vi "HOST_Demodulation_Array.vi"() -> ()   [LabVIEW 2020]
uses:
  <vilib>/rvi/interface/nirviMethod/nirviMethod.xnode
  <vilib>/rvi/errors/niLvFpgaMergeErrorWithErrorCode.vi
  <instrlib>/_niInstr/Streaming/v1/Host/niInstr Streaming v1 Host.lvlib
  <vilib>/rvi/interface/nirviReadWriteControl/nirviReadWriteControl.xnode
  <vilib>/rvi/interface/nirviCloseFPGA/nirviCloseFPGA.xnode
  <vilib>/rvi/interface/nirviOpenFPGA/nirviOpenFPGA.xnode
  <vilib>/rvi/interface/Simulation/niFpgaSimulationCallBeginRW.vi
  <vilib>/rvi/errors/niLvFpgaAdjustHostInterfaceError.vi
  <instrlib>/_niInstr/Streaming/v1/Host/Public/Wait for Stream.vi
  <instrlib>/_niInstr/Streaming/v1/Host/Public/Start Finite Stream.vi
  <instrlib>/_niInstr/Streaming/v1/Host/Public/Start Continuous Stream.vi
  FPGA Bitfiles/rfsignal_FPGATarget_ARRAYCOMPLETECOD_BYxh9E+ljbY.lvbitx
  <vilib>/FPGAPlugInAG/PXIe-7972R/niLvFpga_Open_PXIe-7972R.vi
  <vilib>/rvi/interface/common/dynamic/niFpgaDynamicAddResources.vi
  <vilib>/FPGAPlugInAG/Dynamic/niLvFpga_ConfigureFifo_Dynamic.vi
  <vilib>/FPGAPlugInAG/Dynamic/niLvFpga_StartFifo_Dynamic.vi
  <vilib>/FPGAPlugInAG/Dynamic/niLvFpga_WriteFifo_Dynamic.vi
  <vilib>/FPGAPlugInAG/Dynamic/niLvFpga_Close_Dynamic.vi
  <vilib>/userDefined/Silver/nirio_resource_slv.ctl
  Controls/Clock Select.ctl
panel:
  out "Feedback value check":fxp<+/-,48,32> format="%.26g"
  in  "Decimate AI":u16=100
  in  "CIC length":u16[](array[numeric])
  in  "CIC Cascades":enum16{"1 stage", "2 stage"}(ring)
  in  "Demod Phase 1":u32
  in  "demod":bool
  in  "Modulation":bool[](array[boolean])=[TRUE, FALSE, FALSE, FALSE, FALSE, FALSE, FALSE, FALSE]
  in  "Mod Amp":fxp<+,16,1>[](array[numeric])=[0.5, 1.0, 1.0, 1.0, 0.5, 1.0, 1.0, 1.0]
  in  "Mod Fq (MHz)":dbl[](array[numeric])=[0.1, 1.0, 1.0, 1.0, 0.1, 1.0, 0.0, 1.0] format="%5p"
  in  "stop":bool
  in  "Gain (multiplicative)":fxp<+,32,4>[](array[numeric])=[1.0, 1.0, 1.0, 1.0, 1.0, 1.0, 1.0, 1.0]
  in  "Wave Reader":dbl[](array[numeric])=[27000000.0, 27000000.0, 27000000.0, 27000000.0, 100.0, 27000000.0, 27000000.0, 27000000.0] format="%5p"
  out "AO":waveform(dbl)(graph)={"t0"=timestamp(0.0013999999999999998 s since 1904-01-01), "dt"=3.3333333333333334e-09, "Y"=array[60000 elements]}
  in  "Wave On":bool[](array[boolean])=[FALSE, FALSE, FALSE, FALSE, FALSE, FALSE, FALSE, FALSE]
  in  "Amplitude (V)":dbl[](array[numeric])=[0.33, 0.1, 0.12, 0.12, 0.33, 0.12, 0.12, 0.12] format="%0.2p"
  in  "Frequencies (Hz)":dbl[](array[numeric])=[20000.0, 20000.0, 20000.0, 20000.0, 20000.0, 20000.0, 20000.0, 20000.0] format="%5.0p"
  in  "Signal Type":T1(ring)
  in  "Sampling Info":cluster{"Fs":dbl, "#s":dbl}={"Fs"=300000000.0, "#s"=60000.0} {"Fs" format="%#_3p"}
  out "Error Out":errorcluster
  in  "Update Waveform":bool
  in  "AO Channel":T2(ring)
  in  "Clock Select":T3 items=["Internal Clock", "Internal Clock w/ Ref via CLK/REF IN", "Internal Clock w/ Ref via Sync Clock", "External Clock via CLK/REF IN"]
  in  "Rate of External Sample Clock (MHz)":u16=100 min=60 max=100 step=1
  in  "RIO Resource":T4="RIO0"
  # "Analog In"
  # "Waveform Modification"
  # "Waveform Initialization"
  # "CH1"
  # "Don't change"
  # "CH2"
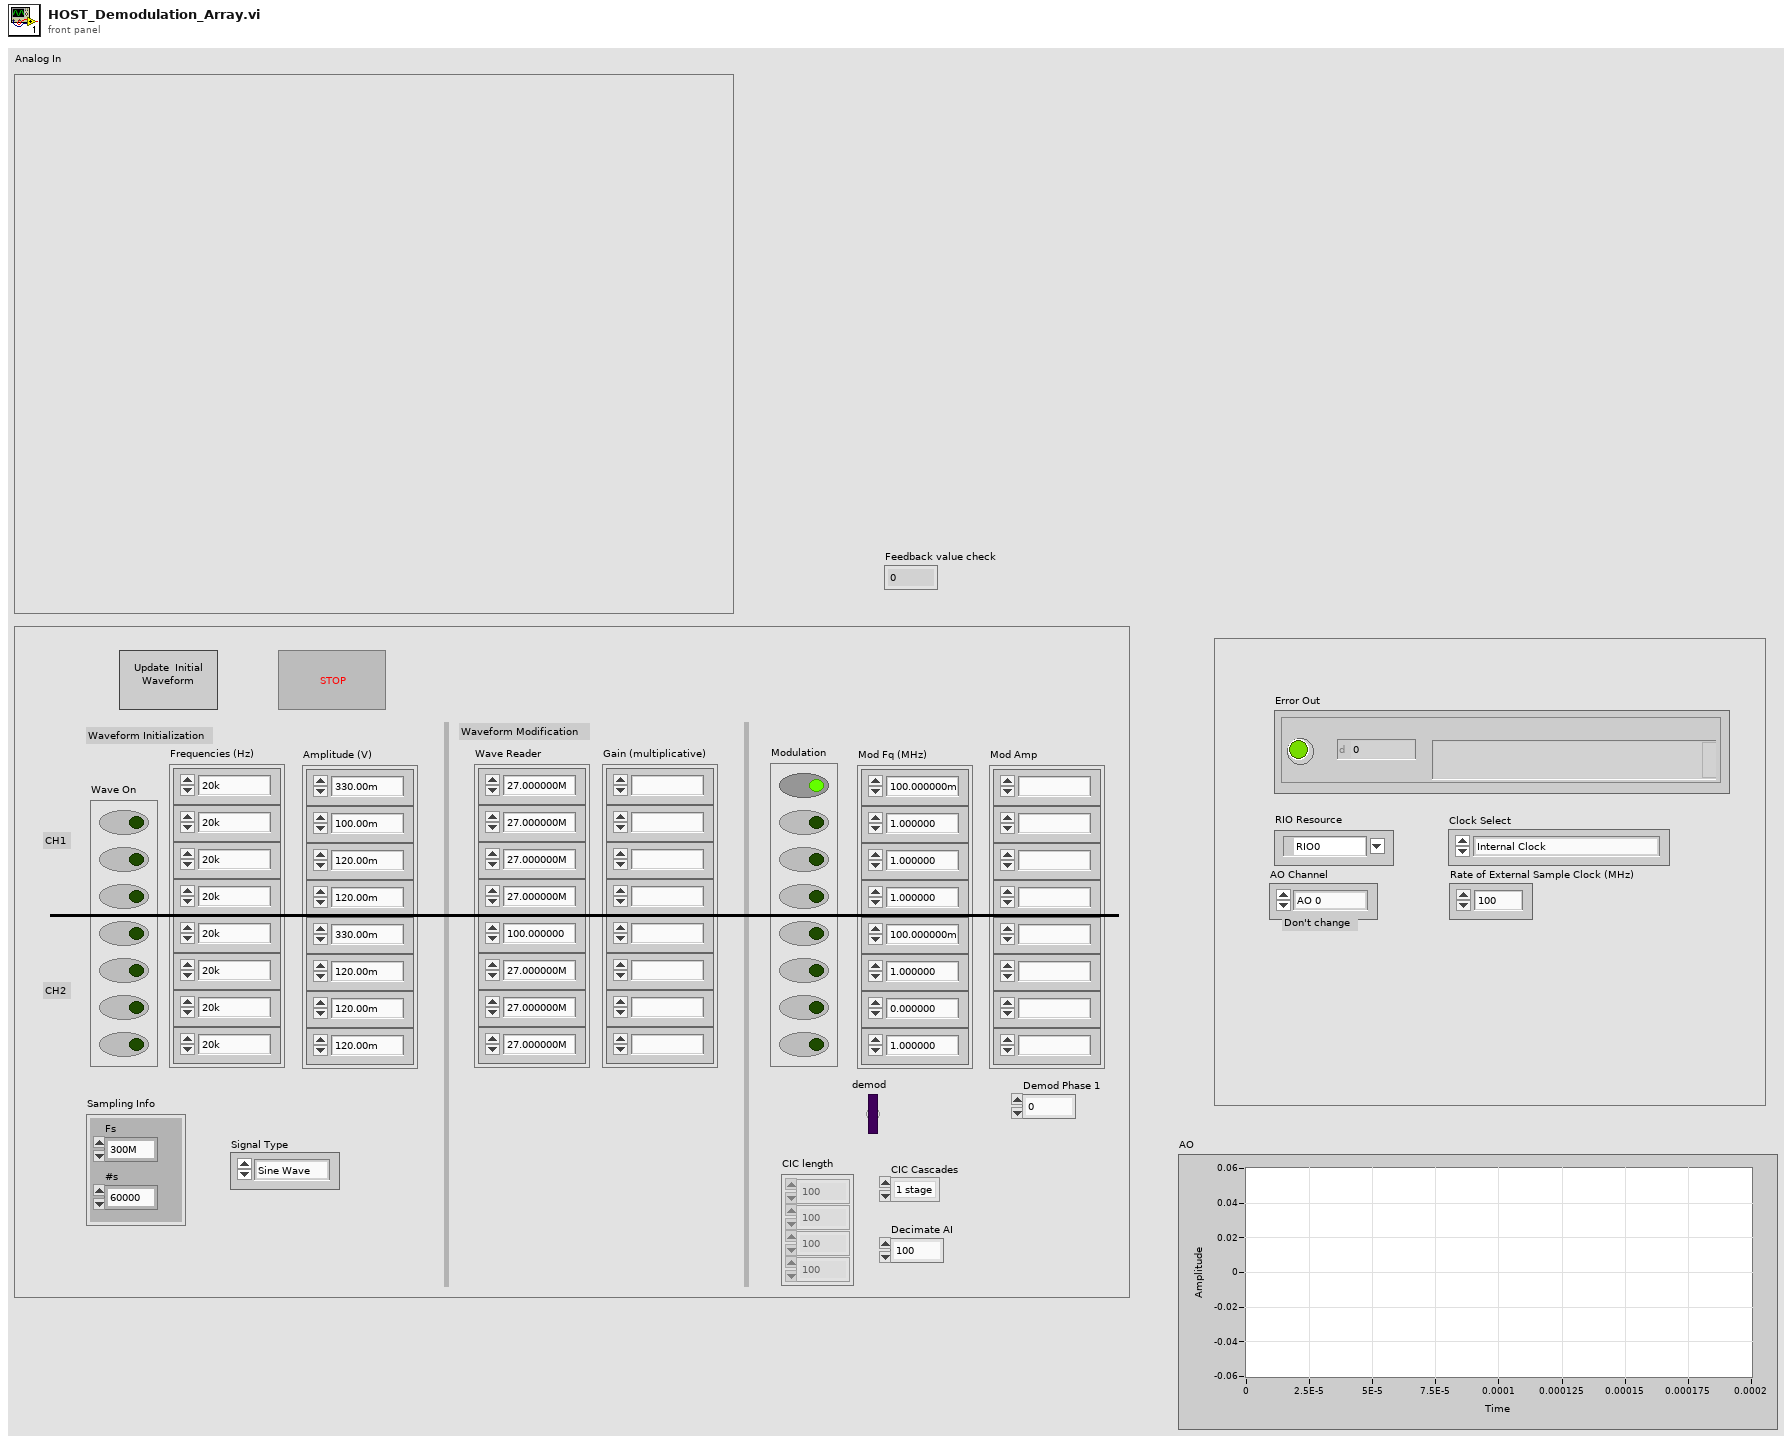
[diagram p1: front panel]
types:
  T1 = enum16{"Sine Wave", "Triangle Wave", "Square Wave", "Sawtooth Wave"}
  T2 = enum8{"AO 0", "AO 1", "AO 2", "AO 3", "AO 0, AO 1, AO 2, AO 3", "None"}
  T3 = typedef "Clock Select.ctl" = u16
  T4 = typedef "nirio_resource_slv.ctl" = tag
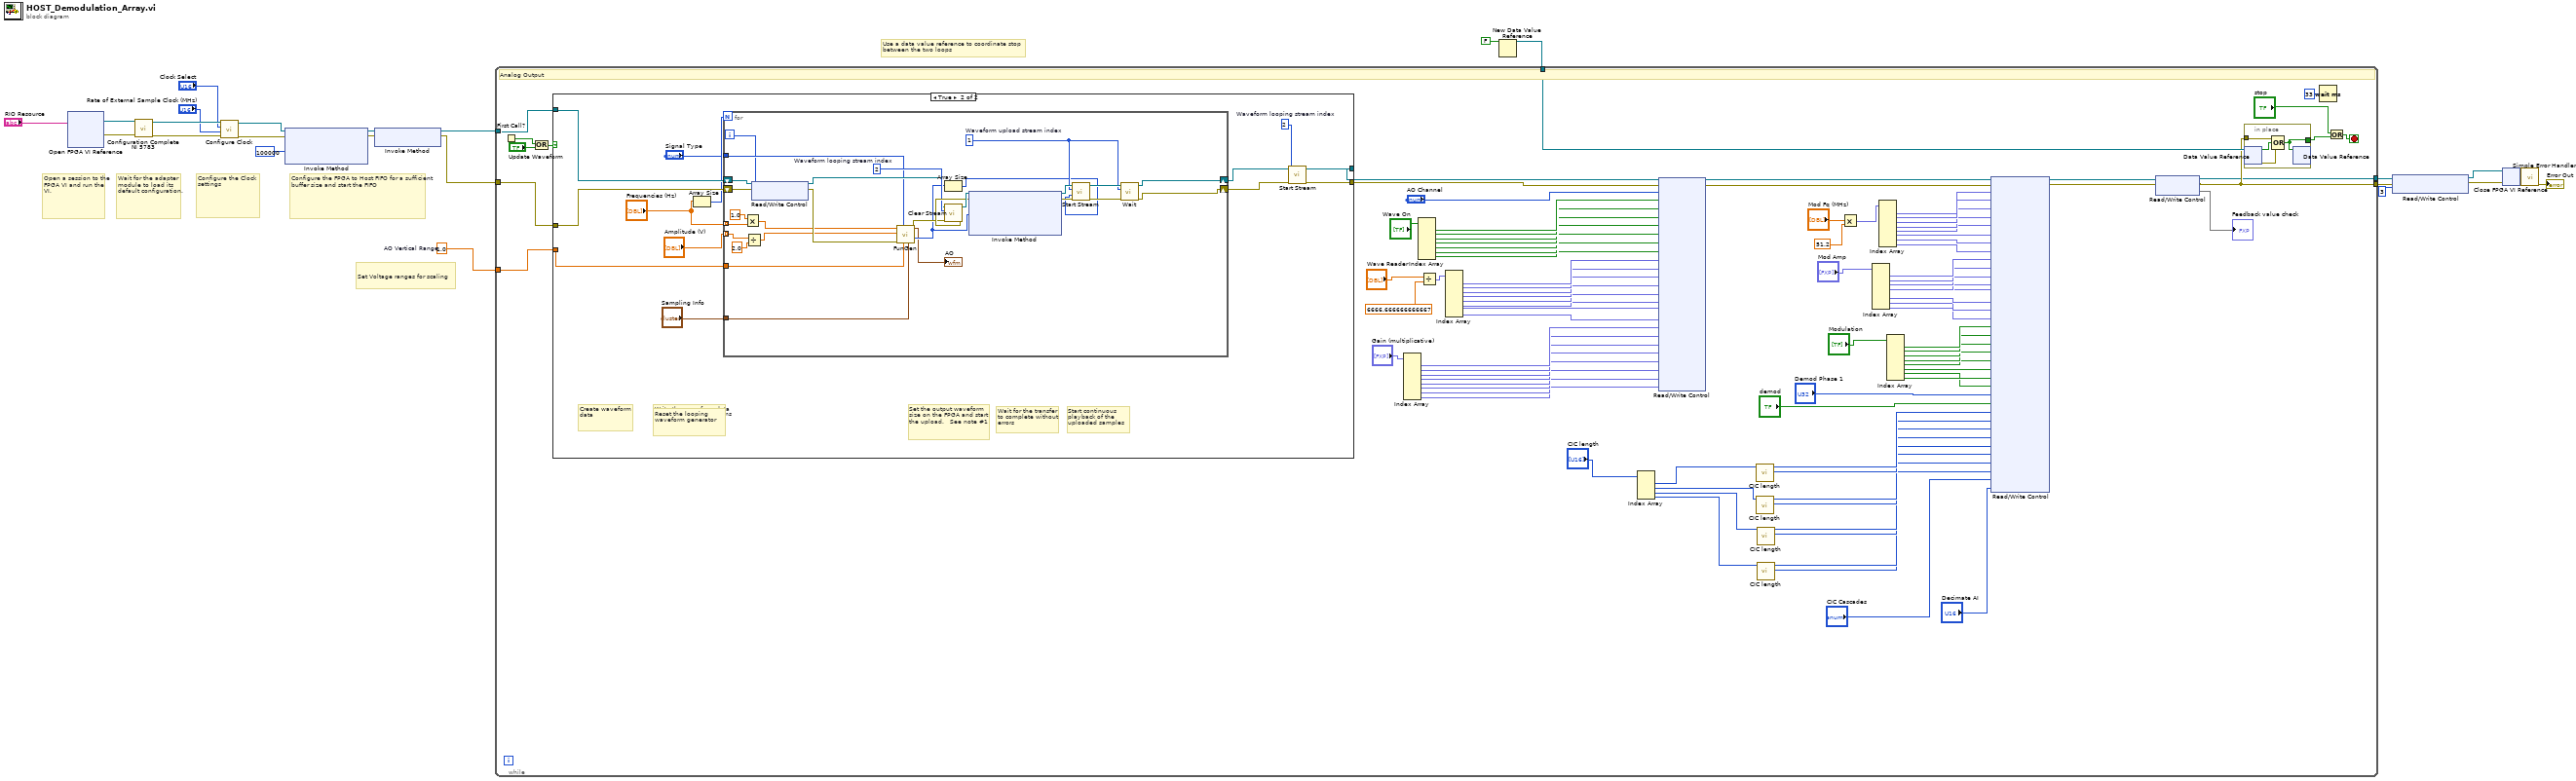
[diagram p0: block diagram]
diagram:
  w12 = 1.0  # AO Vertical Range
  # "Use a data value reference to coordinate stop between the two loops"
  # "Set Voltage ranges for scaling"
  # "Configure the Clock settings"
  # "Configure the FPGA to Host FIFO for a sufficient buffer size and start the FIFO"
  # "Wait for the adapter module to load its default configuration."
  # "Open a session to the FPGA VI and run the VI."
  n1 = xnode "Open FPGA VI Reference"("resource name"="RIO Resource") -> ("FPGA VI Reference Out"=w10:refnum<k20>, "error out"=w9:errorcluster)  [unwired: 1 in]
  n2 = call "Configuration Complete NI 5783.vi"("error in"=w9, "FPGA VI Reference In"=w10) -> ("error out"=w20:errorcluster, "FPGA VI Reference Out"=w21:refnum<k20>)  [unwired: 7 in, 1 out]
  n3 = call "Configure Clock.vi"("error in (no error)"=w20, "Rate of External Sample Clock (MHz)"="Rate of External Sample Clock (MHz)", "Clock Select"="Clock Select", "FPGA VI Reference In"=w21) -> ("error out"=w18:errorcluster, "FPGA VI Reference Out"=w19:refnum<k20>)  [unwired: 3 in, 3 out]
  n4 = xnode "Invoke Method"("FPGA VI Reference In"=w19, "error in"=w18, "Requested Depth"=u32 100000) -> ("FPGA VI Reference Out"=w24:refnum<k20>, "error out"=w23:errorcluster)  [unwired: 1 out]
  n5 = xnode "Invoke Method"("FPGA VI Reference In"=w24, "error in"=w23) -> ("FPGA VI Reference Out"=w3:refnum<k20>, "error out"=w2:errorcluster)
  n6 = New Data Value Reference(data value=FALSE ("Stopped")) -> (data value reference=w1:refnum<data-value>)  [unwired: 1 in, 1 out]
  n7 = while {
    tunnel: w2 -> [w113]
    tunnel: [w28] -> w8
    tunnel: w3 -> [w119]
    tunnel: [w26] -> w7
    tunnel: w1 -> [w114]
    tunnel: w12 -> [w112]
    stop <- w107 stop-if-true
    # "Analog Output"
    n8 = First Call?() -> (First Call?: T/F=w115:bool)
    n9 = Or(x=w115, y="Update Waveform") -> (x .or. y?=w116:bool)
    n10 = case shown="True" w116 {
      tunnel: [w125 w138] -> w111
      tunnel: [w124 w137] -> w110
      tunnel: w119 -> [w125 w135]
      tunnel: w113 -> [w124 w134]
      tunnel: w112 -> [_ w136]
      frame False {
      }
      frame True {
        w133 = 2  # Waveform looping stream index
        # "Loop over the waveforms to combine"
        # "Reset the looping waveform generator"
        # "Start continuous playback of the uploaded samples"
        # "Wait for the transfer to complete without errors"
        # "Set the output waveform size on the FPGA and start the upload.   See note #1"
        # "Write the waveform data to the FPGA for generation"
        # "Create waveform data"
        n11 = Array Size(array="Frequencies (Hz)") -> (size(s)=w128:i32)
        n12 = for {
          N: w128 -> [_]
          tunnel: w136 -> [w156]
          shift-right: [w148] -> w132
          shift-left: w135 -> [w155]
          shift-right: [w147] -> w131
          shift-left: w134 -> [w153]
          tunnel: "Frequencies (Hz)" -> [w146] mode=indexing
          tunnel: "Amplitude (V)" -> [w142] mode=indexing
          tunnel: "Sampling Info" -> [w145]
          tunnel: "Signal Type" -> [w144]
          i -> [w143]
          w157 = 2  # Waveform looping stream index
          w162 = 1  # Waveform upload stream index
          n13 = Multiply(x=1.0, y=w146) -> (x*y=w150:dbl)
          n14 = Divide(x=w142, y=2.0) -> (x/y=w141:dbl)
          n15 = xnode "Read/Write Control"("FPGA VI Reference In"=w155, "error in"=w153, "Upload selector"=w143) -> ("FPGA VI Reference Out"=w154:refnum<k20>, "error out"=w152:errorcluster)
          n16 = call "FunGen.vi"("sampling info"=w145, "range (Vpp)"=w156, "signal type"=w144, "error in (no error)"=w152, "amplitude"=w141, "frequency"=w150) -> ("error out"=w158:errorcluster, "Waveform Data"=w149:i16[], "Output Waveform (V)"=→"AO":waveform(dbl))  [unwired: 2 in, 1 out]
          n17 = Array Size(array=w149) -> (size(s)=w159:i32)
          n18 = call <instrlib>:"Clear Stream.vi"("error in (no error)"=w158, "stream index"=w157, "refnum in"=w154) -> ("error out"=w160:errorcluster, "refnum out"=w161:refnum<k20>)  [unwired: 7 in]
          n19 = xnode "Invoke Method"("FPGA VI Reference In"=w161, "error in"=w160, "Data"=w149) -> ("FPGA VI Reference Out"=w166:refnum<k20>, "error out"=w165:errorcluster)  [unwired: 1 in, 1 out]
          n20 = call-poly <instrlib>:"Start Stream.vi"("error in (no error)"=w165, "num samples"=w159, "stream index"=w162, "refnum in"=w166) -> ("error out"=w163:errorcluster, "refnum out"=w164:refnum<k20>)  [unwired: 6 in]
          n21 = call-poly <instrlib>:"Wait.vi"("error in (no error)"=w163, "stream index"=w162, "refnum in"=w164) -> ("error out"=w147:errorcluster, "refnum out"=w148:refnum<k20>)  [unwired: 5 in, 2 out]
        }
        n22 = call-poly <instrlib>:"Start Stream.vi"("error in (no error)"=w131, "stream index"=w133, "refnum in"=w132) -> ("error out"=w137:errorcluster, "refnum out"=w138:refnum<k20>)  [unwired: 7 in]
      }
    }
    n23 = Index Array(array="Gain (multiplicative)") -> (element #1=w53:fxp<+,32,4>, element #2=w52:fxp<+,32,4>, element #3=w51:fxp<+,32,4>, element #4=w50:fxp<+,32,4>, element #5=w49:fxp<+,32,4>, element #6=w48:fxp<+,32,4>, element #7=w47:fxp<+,32,4>, element #8=w46:fxp<+,32,4>)  [unwired: 8 in]
    n24 = Index Array(array="Wave On") -> (element #1=w68:bool, element #2=w67:bool, element #3=w66:bool, element #4=w65:bool, element #5=w64:bool, element #6=w63:bool, element #7=w62:bool)  [unwired: 7 in]
    n25 = Divide(x="Wave Reader", y=6666.666666666667) -> (x/y=w102:fxp<+,32,16>[])
    n26 = Index Array(array=w102) -> (element #1=w61:fxp<+,32,16>, element #2=w60:fxp<+,32,16>, element #3=w59:fxp<+,32,16>, element #4=w58:fxp<+,32,16>, element #5=w57:fxp<+,32,16>, element #6=w56:fxp<+,32,16>, element #7=w55:fxp<+,32,16>, element #8=w54:fxp<+,32,16>)  [unwired: 8 in]
    n27 = Index Array(array="CIC length") -> (element #1=w34:u16, element #2=w33:u16, element #3=w32:u16, element #4=w35:u16)  [unwired: 4 in]
    n28 = xnode "Read/Write Control"("FPGA VI Reference In"=w111, "error in"=w110, "AO Channel"="AO Channel", "Wave On 2"=w68, "Wave On 3"=w67, "Wave On 4"=w66, "Wave On 5"=w65, "Wave On 6"=w64, "Wave On 7"=w63, "Wave On 8"=w62, "Wave 1"=w61, "Wave 2"=w60, "Wave 3"=w59, "Wave 4"=w58, "Wave 5"=w57, "Wave 6"=w56, "Wave 7"=w55, "Wave 8"=w54, "Amp set 1"=w53, "Amp set 2"=w52, "Amp set 3"=w51, "Amp set 4"=w50, "Amp set 5"=w49, "Amp set 6"=w48, "Amp set 7"=w47, "Amp set 8"=w46) -> ("FPGA VI Reference Out"=w99:refnum<k20>, "error out"=w98:errorcluster)
    n29 = call "CIC length.vi"("CIC total length"=w34) -> ("Length extend"=w43:u8, "CIC length"=w44:u16)  [unwired: 9 in]
    n30 = call "CIC length.vi"("CIC total length"=w33) -> ("Length extend"=w40:u8, "CIC length"=w41:u16)  [unwired: 9 in]
    n31 = call "CIC length.vi"("CIC total length"=w32) -> ("Length extend"=w38:u8, "CIC length"=w39:u16)  [unwired: 9 in]
    n32 = call "CIC length.vi"("CIC total length"=w35) -> ("Length extend"=w36:u8, "CIC length"=w37:u16)  [unwired: 9 in]
    n33 = Multiply(x="Mod Fq (MHz)", y=51.2) -> (x*y=w96:fxp<+,32,13>[])
    n34 = Index Array(array="Mod Amp") -> (element #1=w88:fxp<+,16,1>, element #2=w87:fxp<+,16,1>, element #3=w86:fxp<+,16,1>, element #4=w85:fxp<+,16,1>, element #5=w84:fxp<+,16,1>, element #6=w83:fxp<+,16,1>, element #7=w82:fxp<+,16,1>, element #8=w81:fxp<+,16,1>)  [unwired: 8 in]
    n35 = Index Array(array=w96) -> (element #1=w70:fxp<+,32,13>, element #2=w95:fxp<+,32,13>, element #3=w94:fxp<+,32,13>, element #4=w93:fxp<+,32,13>, element #5=w92:fxp<+,32,13>, element #6=w91:fxp<+,32,13>, element #7=w90:fxp<+,32,13>, element #8=w89:fxp<+,32,13>)  [unwired: 8 in]
    n36 = Index Array(array="Modulation") -> (element #1=w78:bool, element #2=w77:bool, element #3=w76:bool, element #4=w75:bool, element #5=w74:bool, element #6=w73:bool, element #7=w72:bool, element #8=w71:bool)  [unwired: 8 in]
    n37 = xnode "Read/Write Control"("FPGA VI Reference In"=w99, "error in"=w98, "Modulation f 1"=w70, "Modulation f 2"=w95, "Modulation f 3"=w94, "Modulation f 4"=w93, "Modulation f 5"=w92, "Modulation f 6"=w91, "Modulation f 7"=w90, "Modulation f 8"=w89, "Mod amp 1"=w88, "Mod amp 2"=w87, "Mod amp 3"=w86, "Mod amp 4"=w85, "Mod amp 5"=w84, "Mod amp 6"=w83, "Mod amp 7"=w82, "Mod amp 8"=w81, "Modulate 1"=w78, "Modulate 2"=w77, "Modulate 3"=w76, "Modulate 4"=w75, "Modulate 5"=w74, "Modulate 6"=w73, "Modulate 7"=w72, "Modulate 8"=w71, "Demod Phase 1"="Demod Phase 1", "Demod on"="demod", "CIC length 1"=w44, "Length extend 1"=w43, "CIC length 2"=w41, "Length extend 2"=w40, "CIC length 3"=w39, "Length extend 3"=w38, "CIC length 4"=w37, "Length extend 4"=w36, "Stages"="CIC Cascades", "Decimation"="Decimate AI") -> ("FPGA VI Reference Out"=w27:refnum<k20>, "error out"=w29:errorcluster)
    n38 = xnode "Read/Write Control"("FPGA VI Reference In"=w27, "error in"=w29) -> ("FPGA VI Reference Out"=w26:refnum<k20>, "error out"=w28:errorcluster, "Feedback 1"=→"Feedback value check")
    n39 = in-place {
      in-place-border: [w121] -> w106
      in-place-border: w28 -> [w123]
      n40 = in-place-dvr #1(w114) -> (w122:bool, w120:errorcluster)
      n41 = Compound Arithmetic op=OR(w123, w122, w120) -> (w121:bool)
      n42 = in-place-dvr #1(w121) -> ()  [unwired: 2 out]
    }
    n43 = Wait (ms)(milliseconds to wait=u32 33) -> ()  [unwired: 1 out]
    n44 = Or(x="stop", y=w106) -> (x .or. y?=w107:bool)
  }
  n45 = xnode "Read/Write Control"("FPGA VI Reference In"=w7, "error in"=w8, "stream.request state 2"=3) -> ("FPGA VI Reference Out"=w4:refnum<k20>, "error out"=w6:errorcluster)
  n46 = xnode "Close FPGA VI Reference"("FPGA VI Reference In"=w4, "error in"=w6) -> ("error out"=w15:errorcluster)
  n47 = call <vilib>:"Simple Error Handler.vi"("error in (no error)"=w15) -> ("error out"=→"Error Out":errorcluster)  [unwired: 4 in, 4 out]
